vi "Configure Flow Rate Setpoint.vi"(8 "error in (no error)":errorcluster, 10 "flow rate setpoint, calibrated flow unit":dbl, 11 "MKS MF1 in":refnum<class "PL MKS MF1 USB.lvclass">) -> (0 "error out":errorcluster, 3 "MKS MF1 out":refnum<class "PL MKS MF1 USB.lvclass">)   [LabVIEW 2015, in "PL MKS MF1 USB.lvclass"]
doc: "Configures flow rate setpoint."
uses:
  PL MKS MF1 USB.lvclass
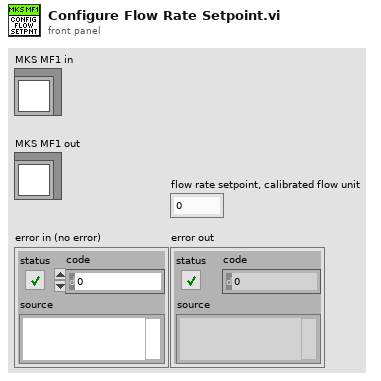
[diagram p1: front panel]
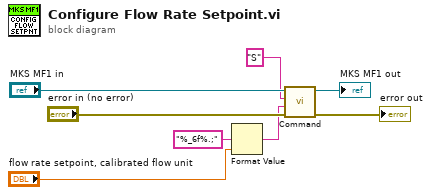
[diagram p0: block diagram]
diagram:
  n1 = Format Value(format string="%_6f%.;", value (0)="flow rate setpoint, calibrated flow unit") -> (output string=w1:string)  [unwired: 1 in]
  n2 = call "Command.vi"("error in (no error)"="error in (no error)", "command value (no value)"=w1, "command"="S", "MKS MF1 in"="MKS MF1 in") -> ("error out"=→"error out":errorcluster, "MKS MF1 out"=→"MKS MF1 out":refnum<class "PL MKS MF1 USB.lvclass">)  [unwired: 4 in, 2 out]
